vi "Set DTRow.vi"(8 "error in (no error)":errorcluster, 10 "Dev Row Elements":string[](array[string])=["", "False", "False", "off.png", "", "Enter a label", "", "", ""], 11 "DevInfo in":refnum<class "DevInfo.lvclass">) -> (0 "error out":errorcluster, 3 "DevInfo out":refnum<class "DevInfo.lvclass">)   [LabVIEW 2016, in "Hardware.lvlib" / "DevInfo.lvclass"]
uses:
  <userlib>/Common Components/Hardware/DevInfo/DevInfo.lvclass
  <userlib>/Common Components/Hardware/DevInfo/DevInfo Cluster Constant.ctl
  <userlib>/Common Components/Hardware/DevInfo/DevInfo.lvclass/DevInfo.ctl
  <vilib>/Utility/error.llb/Error Cluster From Error Code.vi
  <vilib>/ErrorRing/Error Ring.xnode
  <userlib>/LabVIEWdotNetDataGrid/source/DataTable/DataTable.lvclass
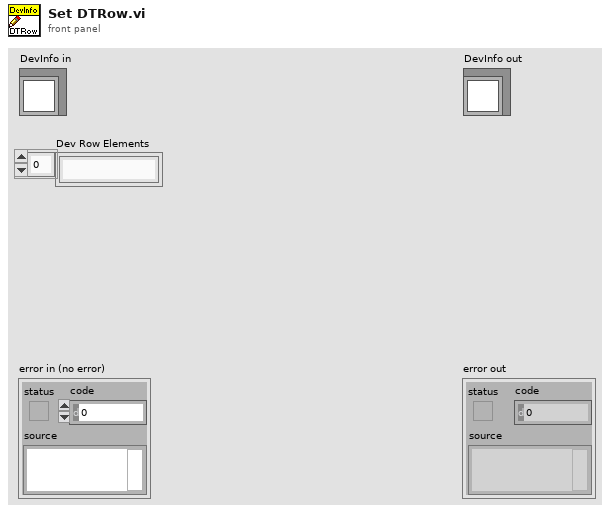
[diagram p1: front panel]
types:
  T1 = typedef "Hardware.lvlib/DevInfo.lvclass/DevInfo Cluster Constant.ctl" = cluster{"GUID":string, "Check":string, "Checked-out":string, "Status":string, "Device":string, "Label":string, "COMM":string, "Sub-COMM":string, "COMM Settings":string}
  T2 = cluster{"Dev Row Elements[0]":string, "Dev Row Elements[1]":string, "Dev Row Elements[2]":string, "Dev Row Elements[3]":string, "Dev Row Elements[4]":string, "Dev Row Elements[5]":string, "Dev Row Elements[6]":string, "Dev Row Elements[7]":string, "Dev Row Elements[8]":string}
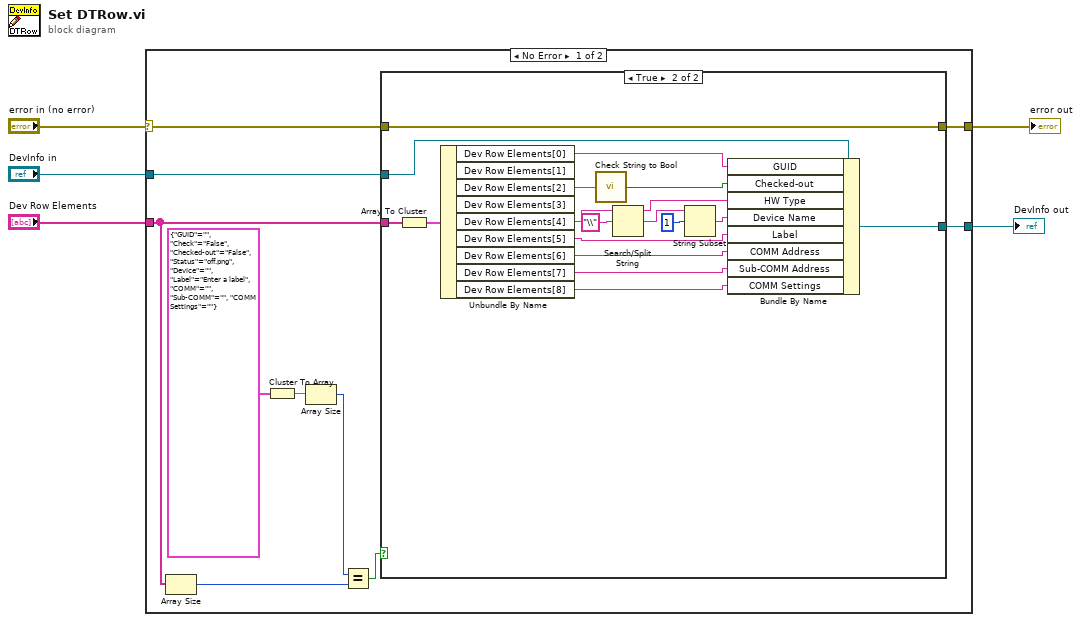
[diagram p0: block diagram]
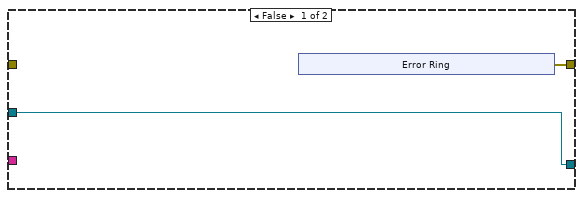
[diagram p2: hidden frame]
diagram:
  n1 = case shown="No Error" "error in (no error)" {
    selector: "error in (no error)" -> [w7 w41]
    tunnel: [w6 w41] -> w4
    tunnel: [w14 w40] -> w2
    tunnel: "DevInfo in" -> [w15 w40]
    tunnel: "Dev Row Elements" -> [w12 _]
    frame No Error {
      n2 = Array Size(array=w12) -> (size(s)=w10:i32)
      n3 = Cluster To Array(cluster=T1 {"GUID"="", "Check"="False", "Checked-out"="False", "Status"="off.png", "Device"="", "Label"="Enter a label", "COMM"="", "Sub-COMM"="", "COMM Settings"=""} ("Cluster")) -> (array=w13:string[])
      n4 = Array Size(array=w13) -> (size(s)=w11:i32)
      n5 = Equal?(x=w11, y=w10) -> (x = y?=w9:bool)
      n6 = case shown="True" w9 {
        tunnel: w15 -> [w17 w39]
        tunnel: [w17 w38] -> w14
        tunnel: w12 -> [_ w36]
        tunnel: w7 -> [_ w24]
        tunnel: [w16 w24] -> w6
        frame False {
          n7 = xnode "Error Ring"() -> ("error out"=w16:errorcluster)
        }
        frame True {
          n8 = Array To Cluster(array=w36) -> (cluster=w37:T2)
          n9 = Unbundle By Name(w37) -> ("Dev Row Elements[0]"=w35:string, "Dev Row Elements[2]"=w34:string, "Dev Row Elements[4]"=w28:string, "Dev Row Elements[5]"=w29:string, "Dev Row Elements[6]"=w30:string, "Dev Row Elements[7]"=w31:string, "Dev Row Elements[8]"=w32:string)  [unwired: 2 out]
          n10 = call <userlib>:"Check String to Bool.vi"("string of check"=w34) -> ("Boolean"=w33:bool)
          n11 = Search/Split String(string=w28, search string/char (-)="\\") -> (substring before match=w26:string, match + rest of string=w25:string)  [unwired: 1 in, 1 out]
          n12 = String Subset(string=w25, offset (0)=1) -> (substring=w23:string)  [unwired: 1 in]
          n13 = Bundle By Name(cluster=w39, "GUID"=w35, "Checked-out"=w33, "HW Type"=w26, "Device Name"=w23, "Label"=w29, "COMM Address"=w30, "Sub-COMM Address"=w31, "COMM Settings"=w32) -> (w38:refnum<class "DevInfo.lvclass">)
        }
      }
    }
    frame Error {
    }
  }
  "error out" <- w4
  "DevInfo out" <- w2
